vi "WS Client Ready.vi"(8 "error in (no error)":errorcluster, 10 "WebSocket Client":refnum<class "WebSocket Client.lvclass">, 11 "Basic WebSocket Manager in":refnum<class "Basic WebSocket Manager.lvclass">) -> (0 "error out":errorcluster)   [LabVIEW 2020, in "HTTP Server.lvlib" / "Basic WebSocket Manager.lvclass"]
uses:
  Basic WebSocket Manager.lvclass
  WebSocket Client/WebSocket Client.lvclass
  Basic WebSocket Manager.lvclass/Basic WebSocket Manager.ctl
  WebSocket Client/WebSocket Client.lvclass/WebSocket Client.ctl
  lv-http-util/HTTP Utils/Request/Request.lvclass/Request.ctl
  lv-uri/URI/URI/URI.lvclass/URI.ctl
  lv-http-util/HTTP Utils/Request/Get Target URI.vi
  lv-uri/URI/URI/Path String.vi
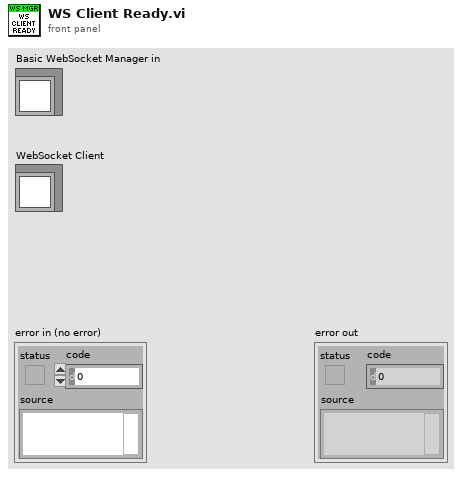
[diagram p1: front panel]
types:
  T1 = cluster{"WebSocket Client":refnum<class "WebSocket Client.lvclass">}
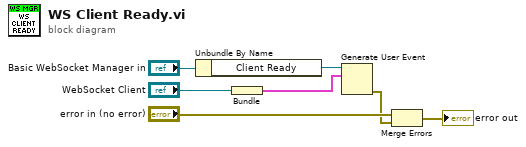
[diagram p0: block diagram]
diagram:
  n1 = Unbundle By Name("Basic WebSocket Manager in") -> ("Client Ready"=w4:refnum<user-event>)
  n2 = Bundle("WebSocket Client"="WebSocket Client") -> (w2:T1)  [unwired: 1 in]
  n3 = Generate User Event(user event=w4, event data cluster=w2) -> (error out=w1:errorcluster)  [unwired: 2 in, 1 out]
  n4 = Merge Errors("error in (no error)", w1) -> (→"error out":errorcluster)
